vi "VelocityConversion.vi"(11 "Velocity (ft/s)":dbl) -> (3 "Velocity (ticks/ds)":dbl)   [LabVIEW 2020]
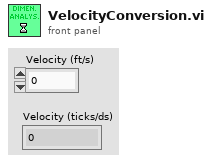
[diagram p1: front panel]
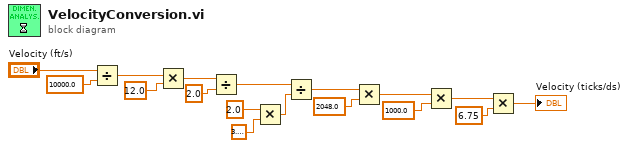
[diagram p0: block diagram]
diagram:
  n1 = Divide(x="Velocity (ft/s)", y=10000.0) -> (x/y=w15:dbl)
  n2 = Multiply(x=w15, y=12.0) -> (x*y=w13:dbl)
  n3 = Divide(x=w13, y=2.0) -> (x/y=w9:dbl)
  n4 = Multiply(x=2.0, y=3.141592653589793) -> (x*y=w8:dbl)
  n5 = Divide(x=w9, y=w8) -> (x/y=w7:dbl)
  n6 = Multiply(x=w7, y=2048.0) -> (x*y=w5:dbl)
  n7 = Multiply(x=w5, y=1000.0) -> (x*y=w3:dbl)
  n8 = Multiply(x=w3, y=6.75) -> (x*y=→"Velocity (ticks/ds)":dbl)
